vi "Zoom.vi"(0 "reference in":refnum<class "LcPictureBox.lvclass">, 2 "ZoomFactor":dbl, 5 "Error In":errorcluster) -> (14 "reference out":refnum<class "LcPictureBox.lvclass">, 15 "ImageUsed":refnum<k24>, 16 "DrawingTime(ms)":u32, 19 "Error Out":errorcluster)   [LabVIEW 2020, in "LcPictureBox.lvclass"]
doc: "Needs to run in User Interface Thread"
uses:
  <userlib>/_LabVIEWCommon/LcPictureBox_class/LcPictureBox.lvclass
  System.Drawing
  System.Windows.Forms
  <userlib>/_LabVIEWCommon/LcPictureBox_class/LcPictureBox.lvclass/LcPictureBox.ctl
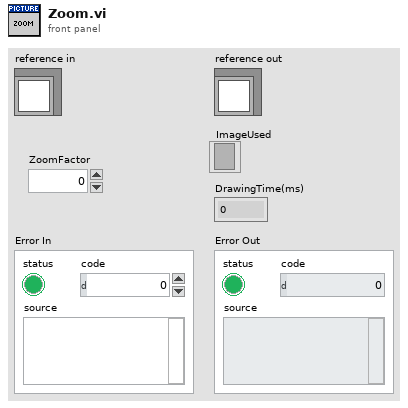
[diagram p1: front panel]
types:
  T1 = typedef "LcPictureBox.lvclass/ObjectAttributes.ctl" = cluster{"PictureBox":refnum<k24>, "ImageSize(PictureBoxSize)":cluster{"Width":i32, "Height":i32}, "PenMemory":map{cluster{"Alpha(100%)":dbl, "Color(Black)":u32, "Pen(Width=1, Solid)":T2}, refnum<k24>}, "GraphicsRef":refnum<k24>, "BrushMemory":map{cluster{"Alpha(100%)":dbl, "Color(Black)":u32}, refnum<k24>}, "Images":refnum<k24>[], "ImageIndex":i32, "BgColor(None)":u32, "LoadedImages":map{string, cluster{"ImageOut":refnum<k24>, "ImageSize":cluster{"Width":i32, "Height":i32}}}}
  T2 = typedef "LcPictureBox.lvclass/Pen.ctl" = cluster{"Width":u16, "Style":enum32{"Solid", "Dash", "Dot", "DashDot", "DashDotDot"}}
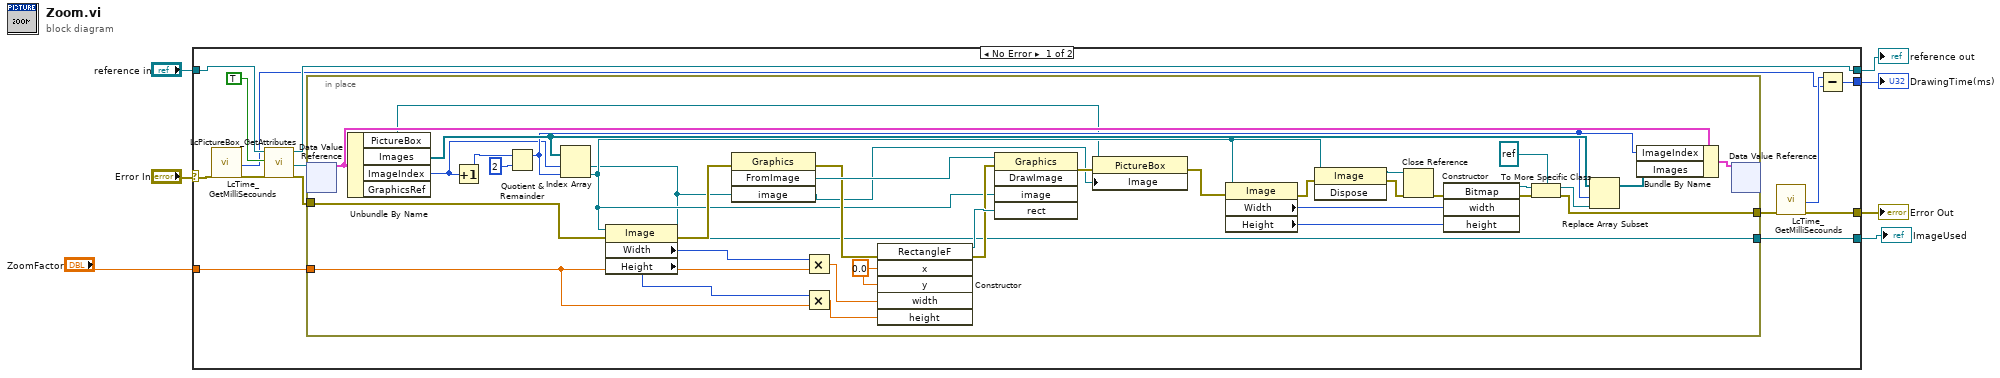
[diagram p0: block diagram]
diagram:
  n1 = case shown="No Error" "Error In" {
    selector: "Error In" -> [w17 w59]
    tunnel: [w14 w59] -> w6
    tunnel: [w21 w58] -> w4
    tunnel: "reference in" -> [w16 w58]
    tunnel: [w10 _] -> w3
    tunnel: [w9 _] -> w2
    tunnel: "ZoomFactor" -> [w8 _]
    frame No Error {
      n2 = call <userlib>:"LcTime_GetMilliSecounds.vi"("error in (no error)"=w17) -> ("msValue"=w11:u32, "error out"=w12:errorcluster)  [unwired: 17 in]
      n3 = call <userlib>:"LcPictureBox_GetAttributes.vi"("reference in"=w16, "OnlyGetDvrReference(False)"=TRUE, "error in (no error)"=w12) -> ("reference out"=w21:refnum<class "LcPictureBox.lvclass">, "DataRef"=w20:refnum<data-value>, "error out"=w18:errorcluster)  [unwired: 13 in, 1 out]
      n4 = in-place {
        in-place-border: w18 -> [w31]
        in-place-border: [w45] -> w15
        in-place-border: [w24] -> w9
        in-place-border: w8 -> [w33]
        w35 = sgl 0.0 ("x")
        n5 = in-place-dvr #1(w20) -> (w57:T1)  [unwired: 1 out]
        n6 = Unbundle By Name(w57) -> ("PictureBox"=w22:refnum<k24>, "Images"=w49:refnum<k24>[], "ImageIndex"=w40:i32)  [unwired: 1 out]
        n7 = Increment(x=w40) -> (x+1=w39:i32)
        n8 = Quotient & Remainder(x=w39, y=2) -> (x-y*floor(x/y)=w48:i32)  [unwired: 1 out]
        n9 = Index Array(array=w49, index #1=w40, index #2=w48) -> (element #1=w24:refnum<k24>, element #2=w25:refnum<k24>)
        n10 = property class="Image"(reference=w25, error in=w31) -> (error out=w32:errorcluster, "Width"=w30:i32, "Height"=w29:i32)  [unwired: 1 out]
        n11 = invoke class="Graphics" method="FromImage"(error in=w32, "image"=w24) -> (error out=w28:errorcluster, "FromImage"=w38:refnum<k24>)  [unwired: 2 in, 2 out]
        n12 = Multiply(x=w30, y=w33) -> (x*y=w36:dbl)
        n13 = Multiply(x=w29, y=w33) -> (x*y=w37:dbl)
        n14 = constructor class="RectangleF"(error in=w28, "x"=w35, "y"=w35, "width"=w36, "height"=w37) -> (reference out=w34:refnum<k24>, error out=w27:errorcluster)  [unwired: 2 in, 5 out]
        n15 = invoke class="Graphics" method="DrawImage"(reference=w38, error in=w27, "image"=w25, "rect"=w34) -> (error out=w26:errorcluster)  [unwired: 1 in, 4 out]
        n16 = property class="PictureBox"(reference=w22, error in=w26, "Image"=w24) -> (error out=w23:errorcluster)  [unwired: 1 out]
        n17 = property class="Image"(reference=w25, error in=w23) -> (error out=w43:errorcluster, "Width"=w51:i32, "Height"=w50:i32)  [unwired: 1 out]
        n18 = invoke class="Image" method="Dispose"(reference=w25, error in=w43) -> (reference out=w41:refnum<k24>, error out=w42:errorcluster)  [unwired: 1 in, 1 out]
        n19 = Close Reference(reference=w41, error in (no error)=w42) -> (error out=w44:errorcluster)
        n20 = constructor class="Bitmap"(error in=w44, "width"=w51, "height"=w50) -> (reference out=w53:refnum<k24>, error out=w52:errorcluster)  [unwired: 2 in, 3 out]
        n21 = To More Specific Class(target class=refnum<k24> refnum, reference=w53, error in=w52) -> (specific class reference=w46:refnum<k24>, error out=w45:errorcluster)
        n22 = Replace Array Subset(array=w49, new element=w46, index=w48) -> (w47:refnum<k24>[])
        n23 = Bundle By Name(cluster=w57, "ImageIndex"=w48, "Images"=w47) -> (w56:T1)
        n24 = in-place-dvr #1(w56) -> ()  [unwired: 2 out]
      }
      n25 = call <userlib>:"LcTime_GetMilliSecounds.vi"("error in (no error)"=w15) -> ("msValue"=w13:u32, "error out"=w14:errorcluster)  [unwired: 17 in]
      n26 = Subtract(x=w13, y=w11) -> (x-y=w10:u32)
    }
    frame Error {
    }
  }
  "Error Out" <- w6
  "reference out" <- w4
  "DrawingTime(ms)" <- w3
  "ImageUsed" <- w2
